vi "EnableDisable Main Page.vi"(8 "error in (no error)":errorcluster, 11 "Node Ptr":u64 format="%.0x") -> (0 "error out":errorcluster)   [LabVIEW 2015, in "Fuel Injector Analysis Addon System Explorer.lvlib"]
uses:
  Fuel Injector Analysis Addon System Explorer.lvlib
  Shared/Constants.vi
  <vilib>/NI VeriStand/Custom Device API/Custom Device API.lvlib
  Shared/Fuel Injector Analysis Addon Shared.lvlib
panel:
  in  "Tag":string
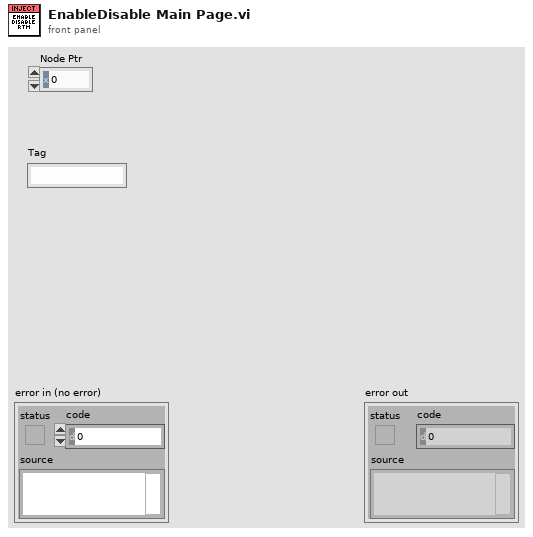
[diagram p1: front panel]
types:
  T1 = typedef "Custom Device API.lvlib/Custom Device Item Ref.ctl" = u64
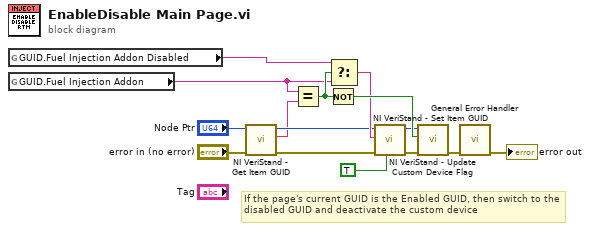
[diagram p0: block diagram]
diagram:
  # "If the page's current GUID is the Enabled GUID, then switch to the disabled GUID and deactivate the custom device"
  n1 = global read "Constants.vi" "GUID.Fuel Injection Addon Disabled"() -> (w1:string)
  n2 = global read "Constants.vi" "GUID.Fuel Injection Addon"() -> (w2:string)
  n3 = call <vilib>:"NI VeriStand - Get Item GUID.vi"("error in (no error)"="error in (no error)", "Item Ref in"="Node Ptr") -> ("error out"=w5:errorcluster, "GUID"=w3:string, "Item Ref out"=w6:T1)  [unwired: 7 in]
  n4 = Equal?(x=w2, y=w3) -> (x = y?=w11:bool)
  n5 = Not(x=w11) -> (.not. x?=w12:bool)
  n6 = Select(t=w1, s=w11, f=w2) -> (s? t:f=w7:string)
  n7 = call <vilib>:"NI VeriStand - Set Item GUID.vi"("Refresh System Explorer Tree? (F)"=TRUE, "error in (no error)"=w5, "GUID"=w7, "Item Ref in"=w6) -> ("error out"=w8:errorcluster, "Item Ref out"=w9:T1)  [unwired: 6 in]
  n8 = call <vilib>:"NI VeriStand - Update Custom Device Flag.vi"("error in (no error)"=w8, "Is Custom Device Active?"=w12, "Device Ref in"=w9) -> ("error out"=w10:errorcluster)  [unwired: 7 in, 1 out]
  n9 = call <vilib>:"General Error Handler.vi"("error in (no error)"=w10) -> ("error out"=→"error out":errorcluster)  [unwired: 10 in, 4 out]
